vi "AddScore.vi"(8 "error in (no error)":errorcluster, 11 "Snake in":refnum<class "Snake.lvclass">) -> (0 "error out":errorcluster, 3 "Snake out":refnum<class "Snake.lvclass">)   [LabVIEW 2019, in "RT_Game.lvlib" / "Snake.lvclass"]
uses:
  Snake.lvclass
  Snake.lvclass/Snake.ctl
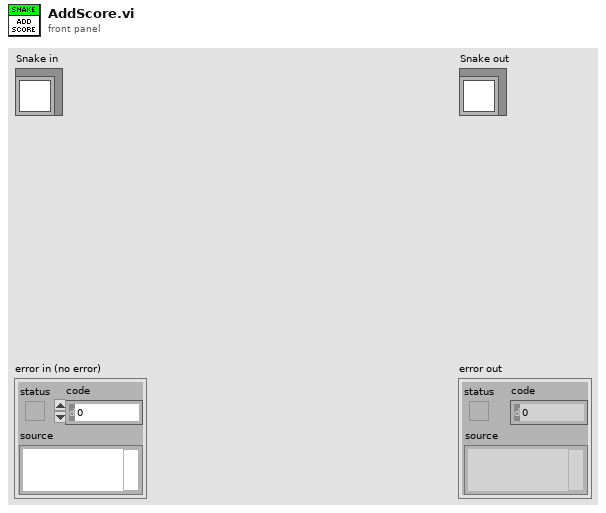
[diagram p1: front panel]
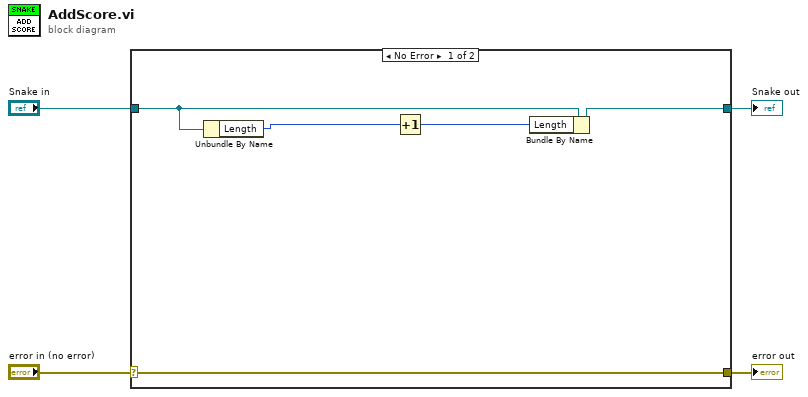
[diagram p0: block diagram]
diagram:
  n1 = case shown="No Error" "error in (no error)" {
    selector: "error in (no error)" -> [w9 w11]
    tunnel: [w9 w11] -> w3
    tunnel: [w8 w10] -> w1
    tunnel: "Snake in" -> [w7 w10]
    frame No Error {
      n2 = Unbundle By Name(w7) -> ("Length"=w6:i16)
      n3 = Increment(x=w6) -> (x+1=w5:i16)
      n4 = Bundle By Name(cluster=w7, "Length"=w5) -> (w8:refnum<class "Snake.lvclass">)
    }
    frame Error {
    }
  }
  "error out" <- w3
  "Snake out" <- w1
